vi "Generic command handler.vi"(8 "error in (no error)":errorcluster, 10 "Message in":refnum<class "GenericMessage.lvclass">, 11 "AOTF in":refnum<class "AOTF.lvclass">) -> (0 "error out":errorcluster, 2 "command":string, 3 "AOTF out":refnum<class "AOTF.lvclass">)   [LabVIEW 2012, in "AOTF.lvclass"]
doc: "The generic_command_handler processes the command 'generic'. Commands which are not part of the predefined list of commands fall under the 'generic' command for special activity."
uses:
  AOTF.lvclass
  <vilib>/Distrio/Murmex/GenericMessage/GenericMessage.lvclass
  <vilib>/Distrio/Murmex/Murmex/Murmex.lvclass
panel:
  # "This method is called when the GENERIC\ntrigger is sent. \n\nOverride this method when your component needs to\nrespond to this trigger. \n\nCall parent for proper implementation"
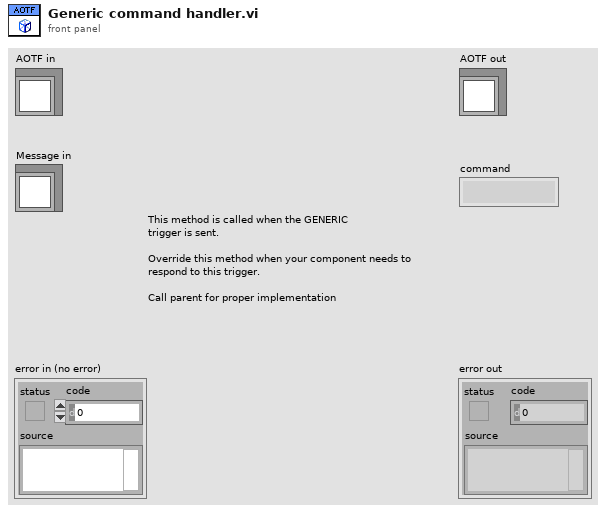
[diagram p1: front panel]
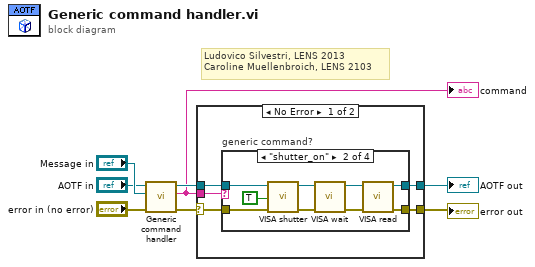
[diagram p0: block diagram]
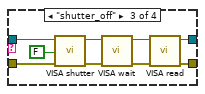
[diagram p3: hidden frame]
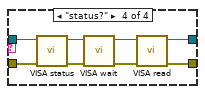
[diagram p4: hidden frame]
diagram:
  # "Ludovico Silvestri, LENS 2013\nCaroline Muellenbroich, LENS 2103"
  n1 = call-parent "Generic command handler.vi"("error in (no error)"="error in (no error)", "Message in"="Message in", "Murmex in"="AOTF in") -> ("error out"=w5:errorcluster, "value"=w1:string, "Murmex out"=w3:refnum<class "AOTF.lvclass">)  [unwired: 6 in]
  "command" <- w1
  n2 = case shown="No Error" w5 {
    selector: w5 -> [w12 w42]
    tunnel: [w13 w42] -> w4
    tunnel: w3 -> [w11 w43]
    tunnel: [w10 w43] -> w2
    tunnel: w1 -> [w9 _]
    frame No Error {
      n3 = case "generic command?" shown="\"shutter_on\"" w9 {
        tunnel: [w14 w19 w28 w35] -> w13
        tunnel: w12 -> [w14 w24 w33 w40]
        tunnel: w11 -> [w15 w23 w32 w41]
        tunnel: [w15 w20 w29 w36] -> w10
        frame Default {
        }
        frame "shutter_on" {
          n4 = call-dynamic "VISA shutter.vi"("error in (no error)"=w24, "button::shutter"=TRUE, "AOTF in"=w23) -> ("error out"=w17:errorcluster, "AOTF out"=w22:refnum<class "AOTF.lvclass">)  [unwired: 7 in]
          n5 = call-dynamic "VISA wait.vi"("error in (no error)"=w17, "AOTF in"=w22) -> ("error out"=w18:errorcluster, "AOTF out"=w21:refnum<class "AOTF.lvclass">)  [unwired: 8 in]
          n6 = call-dynamic "VISA read.vi"("error in (no error)"=w18, "AOTF in"=w21) -> ("error out"=w19:errorcluster, "AOTF out"=w20:refnum<class "AOTF.lvclass">)  [unwired: 7 in, 1 out]
        }
        frame "shutter_off" {
          n7 = call-dynamic "VISA shutter.vi"("error in (no error)"=w33, "button::shutter"=FALSE, "AOTF in"=w32) -> ("error out"=w26:errorcluster, "AOTF out"=w31:refnum<class "AOTF.lvclass">)  [unwired: 7 in]
          n8 = call-dynamic "VISA wait.vi"("error in (no error)"=w26, "AOTF in"=w31) -> ("error out"=w27:errorcluster, "AOTF out"=w30:refnum<class "AOTF.lvclass">)  [unwired: 8 in]
          n9 = call-dynamic "VISA read.vi"("error in (no error)"=w27, "AOTF in"=w30) -> ("error out"=w28:errorcluster, "AOTF out"=w29:refnum<class "AOTF.lvclass">)  [unwired: 7 in, 1 out]
        }
        frame "status?" {
          n10 = call-dynamic "VISA status.vi"("error in (no error)"=w40, "AOTF in"=w41) -> ("error out"=w38:errorcluster, "AOTF out"=w39:refnum<class "AOTF.lvclass">)  [unwired: 8 in]
          n11 = call-dynamic "VISA wait.vi"("error in (no error)"=w38, "AOTF in"=w39) -> ("error out"=w34:errorcluster, "AOTF out"=w37:refnum<class "AOTF.lvclass">)  [unwired: 8 in]
          n12 = call-dynamic "VISA read.vi"("error in (no error)"=w34, "AOTF in"=w37) -> ("error out"=w35:errorcluster, "AOTF out"=w36:refnum<class "AOTF.lvclass">)  [unwired: 7 in, 1 out]
        }
      }
    }
    frame Error {
    }
  }
  "error out" <- w4
  "AOTF out" <- w2
